vi "Configure Instrument.vi"(0 "Instrument Handle In":refnum<k21>, 5 "Instrument Configuration":T1={"LO Sharing Mode"=enum."Automatic", "Frequency Reference Source"="PXI_Clk"}, 11 "error in (no error)":errorcluster) -> (4 "Instrument Handle Out":refnum<k21>, 15 "error out":errorcluster)   [LabVIEW 2019, in "RFmxInstr.lvlib"]
doc: "Applies common instrument settings to the analyzer."
uses:
  RFmxInstr.lvlib
  Typedefs/Instrument Configuration.ctl
  Common/Local Oscillator Sharing Mode.ctl
  <resource>/objmgr/RFmxInstr.rc
  Common/Common.lvlib
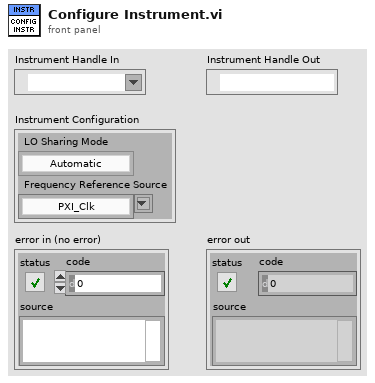
[diagram p1: front panel]
types:
  T1 = typedef "RFmxInstr.lvlib/Instrument Configuration.ctl" = cluster{"LO Sharing Mode":T2, "Frequency Reference Source":string}
  T2 = typedef "Common.lvlib/Local Oscillator Sharing Mode.ctl" = enum16{"Automatic", "None"}
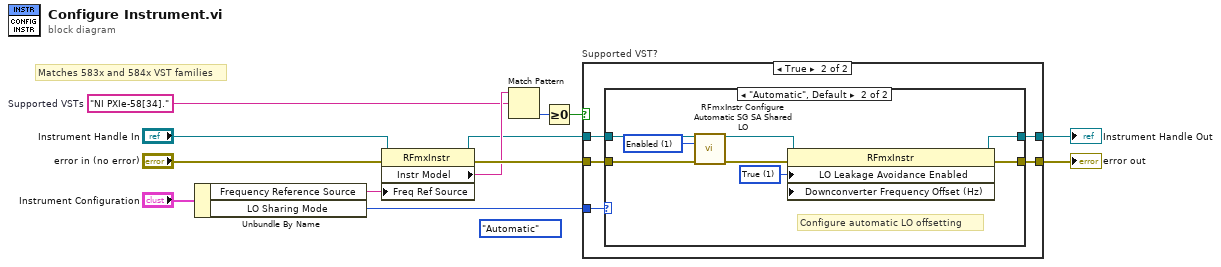
[diagram p0: block diagram]
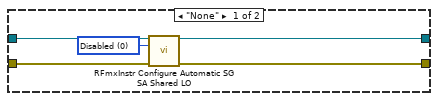
[diagram p3: hidden frame]
diagram:
  (unwired) Local_Oscillator_Sharing_Mode."Automatic" ("LO Sharing Mode")
  w10 = "NI PXIe-58[34]."  # Supported VSTs
  # "Matches 583x and 584x VST families"
  n1 = Unbundle By Name("Instrument Configuration") -> ("Frequency Reference Source"=w1:string, "LO Sharing Mode"=w2:T2)
  n2 = property class="RFmxInstr"(reference="Instrument Handle In", error in="error in (no error)", "Freq Ref Source"=w1) -> (reference out=w6:refnum<k21>, error out=w13:errorcluster, "Instr Model"=w11:string)
  n3 = Match Pattern(string=w11, regular expression=w10) -> (offset past match=w9:i32)  [unwired: 1 in, 3 out]
  n4 = Greater Or Equal To 0?(x=w9) -> (x >= 0?=w4:bool)
  n5 = case "Supported VST?" shown="True" w4 {
    tunnel: [w15 w19] -> w8
    tunnel: w13 -> [w14 w16]
    tunnel: [w14 w20] -> w7
    tunnel: w6 -> [w15 w17]
    tunnel: w2 -> [_ w18]
    frame False {
      # "Do nothing; any configuration for LOs with standalone VSAs should be configured manually. Baseband instruments don't have LOs. Unsupported VSTs must be configured manually."
    }
    frame True {
      n6 = case shown="\"Automatic\", Default" w18 {
        tunnel: [w22 w33] -> w20
        tunnel: [w23 w26] -> w19
        tunnel: w17 -> [w25 w31]
        tunnel: w16 -> [w24 w30]
        frame "None" {
          w21 = 0 items=["Disabled", "Enabled"] ("Automatic SG SA Shared LO")
          n7 = call <vilib>:"RFmxInstr Configure Automatic SG SA Shared LO.vi"("Instrument Handle In"=w25, "Automatic SG SA Shared LO"=w21, "error in (no error)"=w24) -> ("Instrument Handle Out"=w23:refnum<k21>, "error out"=w22:errorcluster)  [unwired: 11 in]
        }
        frame "Automatic", Default {
          w27 = 1 items=["Disabled", "Enabled"] ("Automatic SG SA Shared LO")
          w32 = 1 items=["False", "True"] ("LO Leakage Avoidance Enabled")
          # "Configure automatic LO offsetting"
          n8 = call <vilib>:"RFmxInstr Configure Automatic SG SA Shared LO.vi"("Instrument Handle In"=w31, "Automatic SG SA Shared LO"=w27, "error in (no error)"=w30) -> ("Instrument Handle Out"=w28:refnum<k21>, "error out"=w29:errorcluster)  [unwired: 11 in]
          n9 = property class="RFmxInstr" props=["LO Leakage Avoidance Enabled", "Downconverter Frequency Offset (Hz)"](reference=w28, error in=w29, "LO Leakage Avoidance Enabled"=w32) -> (reference out=w26:refnum<k21>, error out=w33:errorcluster)  [unwired: 1 in]
        }
      }
    }
  }
  "error out" <- w7
  "Instrument Handle Out" <- w8
